vi "Add Status Channel to All Transfers.vi"(7 "GUID (Default Channel)":string="03D3BB99-1485-13A6-561D1F898F032919", 8 "error in (no error)":errorcluster, 9 "Channel":T1, 10 "Channel Name":string, 11 "Item Ref in":T3 format="%.0x") -> (0 "error out":errorcluster, 3 "Item Ref out":T3 format="%.0x")   [LabVIEW 2017, in "DSF System Explorer.lvlib"]
uses:
  DSF System Explorer.lvlib
  <vilib>/NI Veristand/Custom Device API/Custom Device Item Ref.ctl
  <vilib>/NI Veristand/Custom Device API/Custom Device Channel.ctl
  <vilib>/NI Veristand/Custom Device API/Custom Device Channel Type.ctl
  <vilib>/NI Veristand/Custom Device API/Custom Device API.lvlib
  Shared/DSF Shared.lvlib
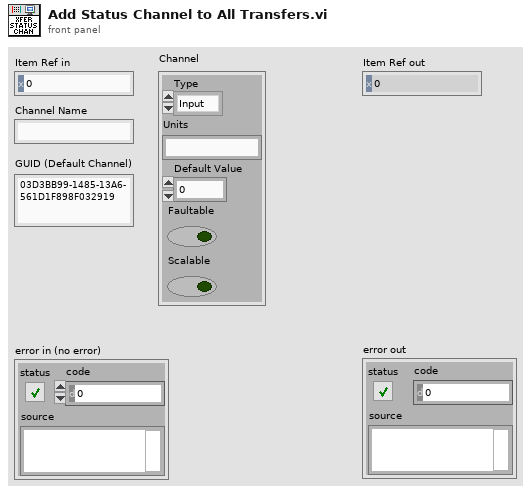
[diagram p1: front panel]
types:
  T1 = typedef "Custom Device API.lvlib/Custom Device Channel.ctl" = cluster{"Type":T2, "Units":string, "Default Value":dbl, "Faultable":bool, "Scalable":bool}
  T2 = typedef "Custom Device API.lvlib/Custom Device Channel Type.ctl" = enum16{"Input", "Output"}
  T3 = typedef "Custom Device API.lvlib/Custom Device Item Ref.ctl" = u64
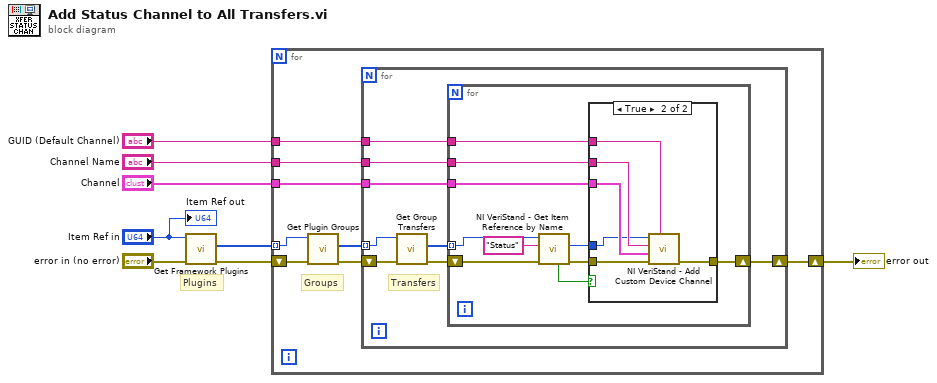
[diagram p0: block diagram]
diagram:
  # "Plugins"
  n1 = call "Get Framework Plugins.vi"("error in (no error)"="error in (no error)", "Framework Ref in"="Item Ref in") -> ("error out"=w6:errorcluster, "Plugin refs"=w5:T3[])  [unwired: 7 in, 1 out]
  n2 = for {
    shift-right: [w13] -> w4
    shift-left: w6 -> [w16]
    tunnel: w5 -> [w15] mode=indexing
    tunnel: "Channel Name" -> [w11]
    tunnel: "Channel" -> [w10]
    tunnel: "GUID (Default Channel)" -> [w9]
    # "Groups"
    n3 = call "Get Plugin Groups.vi"("error in (no error)"=w16, "Plugin Ref in"=w15) -> ("error out"=w14:errorcluster, "Group refs"=w12:T3[])  [unwired: 7 in, 1 out]
    n4 = for {
      shift-right: [w24] -> w13
      shift-left: w14 -> [w23]
      tunnel: w12 -> [w21] mode=indexing
      tunnel: w11 -> [w20]
      tunnel: w10 -> [w17]
      tunnel: w9 -> [w19]
      # "Transfers"
      n5 = call "Get Group Transfers.vi"("error in (no error)"=w23, "Group Ref in"=w21) -> ("error out"=w22:errorcluster, "Transfer refs"=w18:T3[])  [unwired: 7 in, 1 out]
      n6 = for {
        shift-right: [w28] -> w24
        shift-left: w22 -> [w30]
        tunnel: w17 -> [w27]
        tunnel: w20 -> [w26]
        tunnel: w19 -> [w25]
        tunnel: w18 -> [w29] mode=indexing
        n7 = call <vilib>:"NI VeriStand - Get Item Reference by Name.vi"("error in (no error)"=w30, "Item Name"="Status", "Parent Ref in"=w29) -> ("error out"=w32:errorcluster, "Item Ref"=w31:T3, "Found"=w33:bool)  [unwired: 5 in, 1 out]
        n8 = case shown="True" w33 {
          tunnel: w32 -> [w35 w41]
          tunnel: w31 -> [_ w37]
          tunnel: [w35 w36] -> w28
          tunnel: w27 -> [_ w40]
          tunnel: w26 -> [_ w39]
          tunnel: w25 -> [_ w38]
          frame False {
          }
          frame True {
            n9 = call <vilib>:"NI VeriStand - Add Custom Device Channel.vi"("GUID (Default Channel)"=w38, "error in (no error)"=w41, "Channel"=w40, "Channel Name"=w39, "Parent Ref in"=w37) -> ("error out"=w36:errorcluster)  [unwired: 3 in, 3 out]
          }
        }
      }
    }
  }
  "error out" <- w4
  "Item Ref out" <- "Item Ref in"
